vi "3. Rotate in any direction.vi"() -> ()   [LabVIEW 2020]
uses:
  <vilib>/robotics/Starter Kit/2.0/9632 Host Interface/NI_Robotics_Starter Kit Host_9632_2.0.lvclass
panel:
  out "Waveform Chart":cluster{dbl, dbl}(graph)
  in  "Rotation degree":dbl(knob) scale=0.0..360.0
  in  "Robot Velocity":dbl(slide) scale=0.0..0.3
  in  "Action":T1(ring)
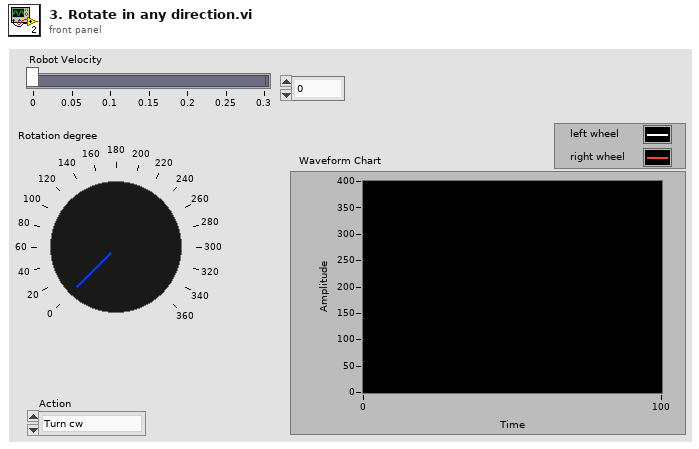
[diagram p1: front panel]
types:
  T1 = enum16{"Turn cw", "Turn ccw", "Rotate cw", "Rotate ccw"}
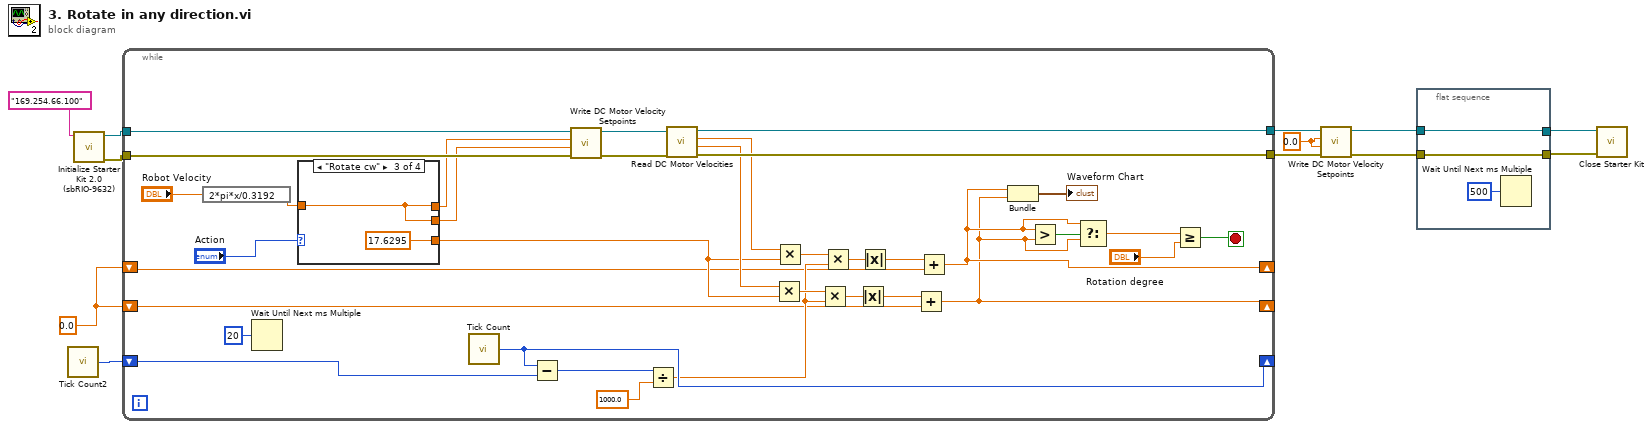
[diagram p0: block diagram]
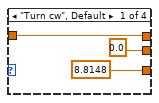
[diagram p2: hidden frame]
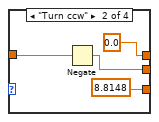
[diagram p3: hidden frame]
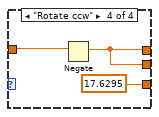
[diagram p4: hidden frame]
diagram:
  w3 = 0.0 ("left motor ccw velocity (rad/s)")
  w8 = 0.0 ("y")
  n1 = call "Tick Count2"() -> ("Tick Count(mSec)"=w9:u32)
  n2 = call <vilib>:"Initialize Starter Kit 2.0 (sbRIO-9632).vi"("IP address (\"\")"="169.254.66.100" ("IP address (\"\")")) -> ("error out"=w10:errorcluster, "FPGA starter kit host 2.0 out"=w11:refnum<class "NI_Robotics_Starter Kit Host_9632_2.0.lvclass">)  [unwired: 9 in]
  n3 = while {
    tunnel: w11 -> [w47]
    tunnel: w10 -> [w46]
    tunnel: [w43] -> w7
    tunnel: [w42] -> w6
    shift-right: [w28] -> _
    shift-left: w9 -> [w39]
    shift-right: [w18] -> _
    shift-left: w8 -> [w21]
    shift-right: [w17] -> _
    shift-left: w8 -> [w22]
    stop <- w14 stop-if-true
    n4 = expression code="2*pi*x/0.3192" ("RPM to radian/s")("Robot Velocity") -> (w34:dbl)
    n5 = Wait Until Next ms Multiple(millisecond multiple=u32 20) -> ()  [unwired: 1 out]
    n6 = case shown="\"Rotate cw\"" "Action" {
      tunnel: [w49 0.0 ("y") w55 w57] -> w38
      tunnel: [0.0 ("y") w52 w55 w57] -> w37
      tunnel: [8.8148 ("y") 8.8148 ("y") 17.6295 ("y") 17.6295 ("y")] -> w31
      tunnel: w34 -> [w49 w54 w55 w59]
      frame "Turn cw", Default {
      }
      frame "Turn ccw" {
        n7 = Negate(x=w54) -> (-x=w52:dbl)
      }
      frame "Rotate cw" {
      }
      frame "Rotate ccw" {
        n8 = Negate(x=w59) -> (-x=w57:dbl)
      }
    }
    n9 = call "Tick Count"() -> ("Tick Count(mSec)"=w28:u32)
    n10 = Subtract(x=w28, y=w39) -> (x-y=w41:u32)
    n11 = call <vilib>:"Write DC Motor Velocity Setpoints.vi"("error in (no error)"=w46, "right motor ccw velocity (rad/s)"=w37, "left motor ccw velocity (rad/s)"=w38, "starter kit host in"=w47) -> ("error out"=w44:errorcluster, "starter kit host out"=w45:refnum<class "NI_Robotics_Starter Kit Host_9632_2.0.lvclass">)  [unwired: 6 in]
    n12 = Divide(x=w41, y=1000.0) -> (x/y=w27:dbl)
    n13 = call <vilib>:"Read DC Motor Velocities.vi"("error in (no error)"=w44, "starter kit host in"=w45) -> ("error out"=w42:errorcluster, "right motor ccw velocity (rad/s)"=w32:dbl, "left motor ccw velocity (rad/s)"=w33:dbl, "starter kit host out"=w43:refnum<class "NI_Robotics_Starter Kit Host_9632_2.0.lvclass">)  [unwired: 6 in]
    n14 = Multiply(x=w32, y=w31) -> (x*y=w29:dbl)
    n15 = Multiply(x=w33, y=w31) -> (x*y=w30:dbl)
    n16 = Multiply(x=w29, y=w27) -> (x*y=w25:dbl)
    n17 = Multiply(x=w30, y=w27) -> (x*y=w26:dbl)
    n18 = Absolute Value(x=w25) -> (abs(x)=w23:dbl)
    n19 = Absolute Value(x=w26) -> (abs(x)=w24:dbl)
    n20 = Add(x=w23, y=w22) -> (x+y=w17:dbl)
    n21 = Add(x=w24, y=w21) -> (x+y=w18:dbl)
    n22 = Bundle(w18, w17) -> (→"Waveform Chart":cluster{dbl, dbl})  [unwired: 1 in]
    n23 = Greater?(x=w18, y=w17) -> (0:w19:bool)
    n24 = Select(t=w18, s=w19, f=w17) -> (s? t:f=w16:dbl)
    n25 = Greater Or Equal?(x=w16, y="Rotation degree") -> (x >= y?=w14:bool)
  }
  n26 = call <vilib>:"Write DC Motor Velocity Setpoints.vi"("error in (no error)"=w6, "right motor ccw velocity (rad/s)"=w3, "left motor ccw velocity (rad/s)"=w3, "starter kit host in"=w7) -> ("error out"=w4:errorcluster, "starter kit host out"=w5:refnum<class "NI_Robotics_Starter Kit Host_9632_2.0.lvclass">)  [unwired: 6 in]
  n27 = flat-sequence {
    tunnel: w5 -> [w62]
    tunnel: w4 -> [w61]
    tunnel: [w62] -> w2
    tunnel: [w61] -> w1
    frame #0 {
      n28 = Wait Until Next ms Multiple(millisecond multiple=u32 500) -> ()  [unwired: 1 out]
    }
  }
  n29 = call-dynamic "Close Starter Kit.vi"("error in (no error)"=w1, "starter kit host in"=w2) -> ()  [unwired: 9 in, 1 out]
